vi "S3 Tool Initial.vi"() -> (0 "error constant":errorcluster)   [LabVIEW 2019]
uses:
  Ctrl/StationCmdSelect.ctl
  Ctrl/Auto Inspection Station Name2.ctl
  Ctrl/Auto Inspection Data Name.ctl
  Global/Process Global.vi
  LineScan/LineScan.lvclass
  LLB/Commonly VI.lvlib
panel:
  out "ToolStringOut_Init":string
  out "Initial_ChkSum":string
  out "S3 Initial Status":bool
  out "Initial receive":string
  out "retry次數 2":string[](array[string])
  out "CurrentCmd 2":string
  out "Retry 2":i32
  in  "Numeric 3":i32
  out "Act Step":i32
  out "Numeric":dbl
  out "subarray":string[](array[string])
  in  "error in (no error) 2":errorcluster
  out "retry次數":string[](array[string])
  out "CurrentCmd":string
  out "Retry":i32
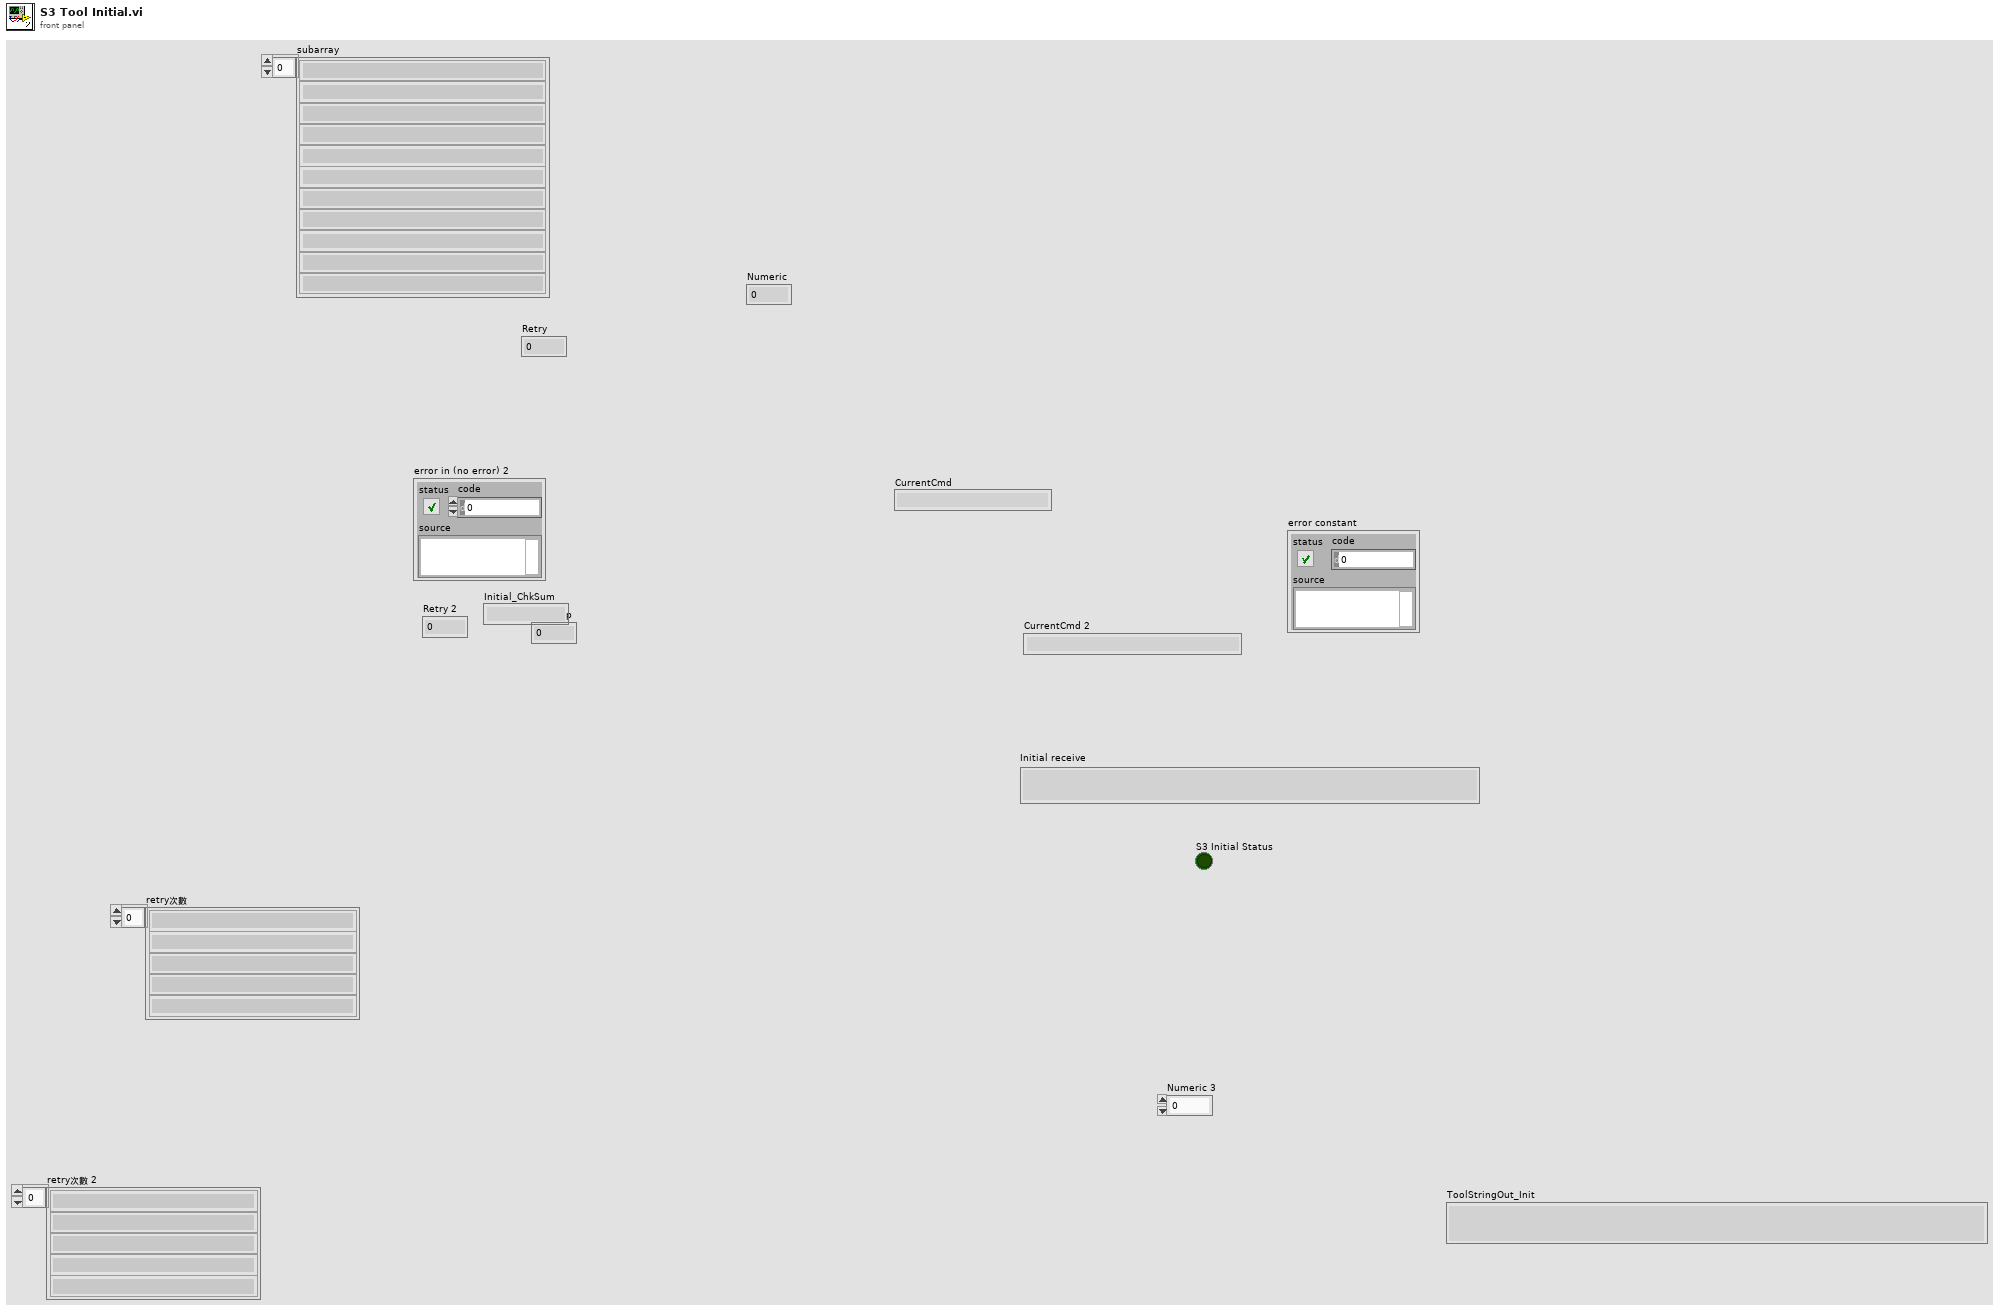
[diagram p1: front panel]
types:
  T1 = typedef "StationCmdSelect.ctl" = enum16{"Action", "Command", "Return", "DTime", "Retry"}
  T2 = typedef "Auto Inspection Data Name.ctl" = enum16{"LocalRun", "ItemSN(TimeCode)", "CurrentAction", "Error", "Data", "OKNG", "電壓值", "電壓值判斷", "電流值", "電流值判斷", "Laser1 Data", "Laser2 Data", "Laser OKNG", "StationNO"}
  T3 = typedef "Auto Inspection Station Name2.ctl" = enum16{"S1Barcode", "S2Measure", "S3Measure", "S4Measure", "S5Measure", "S11_LaserCheck", "S8_Vision AI"}
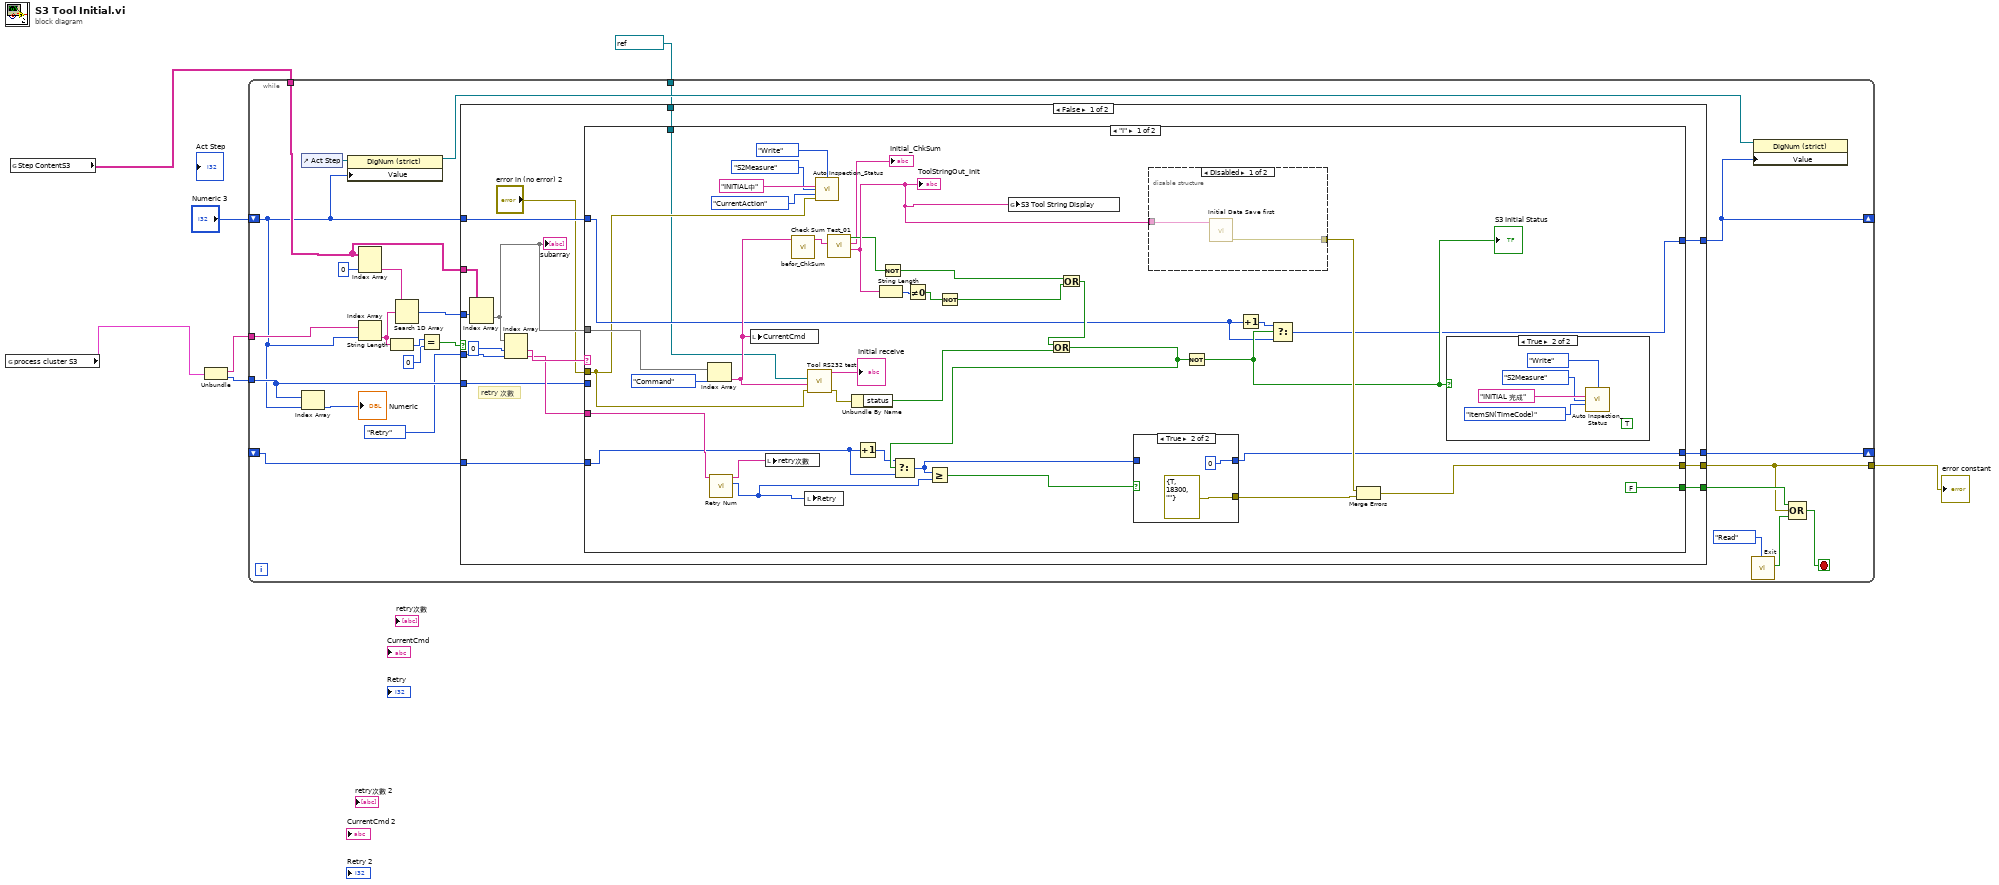
[diagram p0: block diagram]
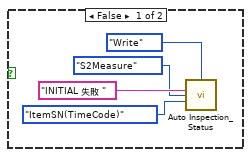
[diagram p3: hidden frame]
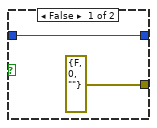
[diagram p4: hidden frame]
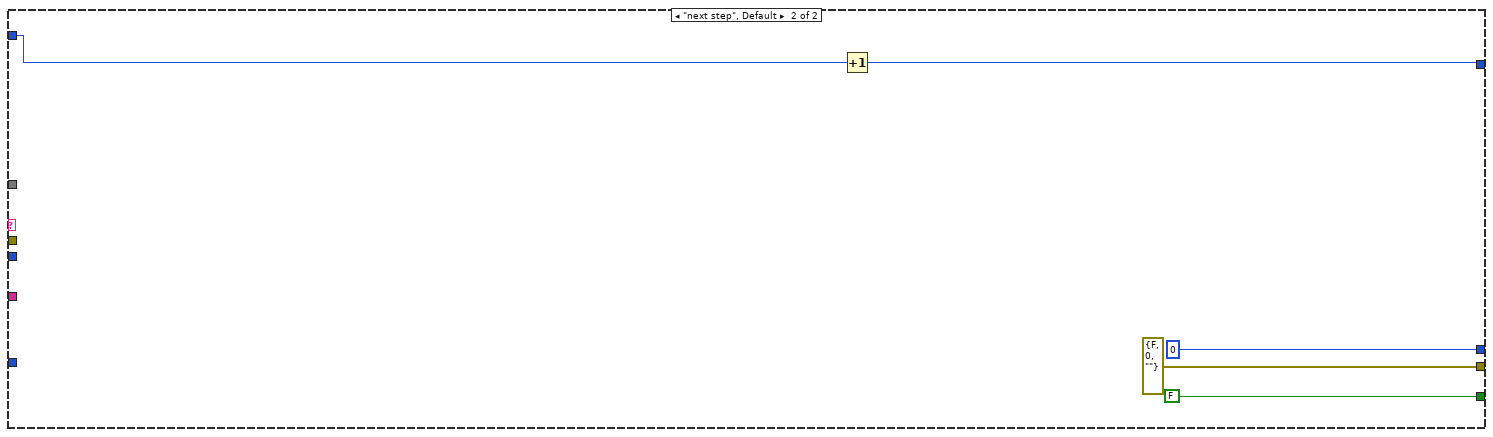
[diagram p5: hidden frame]
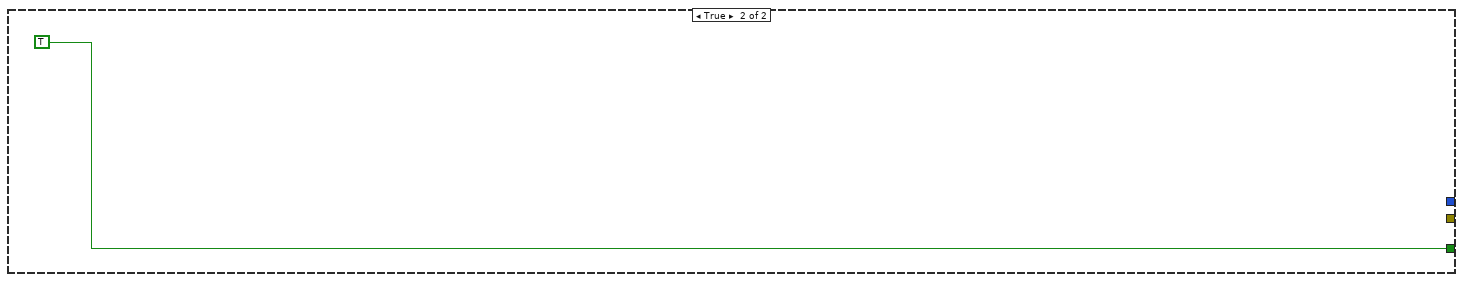
[diagram p6: hidden frame]
diagram:
  n1 = global read "Process Global.vi" "process cluster S3"() -> (w2:cluster{string[], i32[]})
  n2 = global read "Process Global.vi" "Step ContentS3"() -> (w3:string[][])
  n3 = Unbundle(w2) -> (w7:string[], w6:i32[])
  n4 = while {
    tunnel: w7 -> [w31]
    tunnel: w6 -> [w30]
    tunnel: w3 -> [w29]
    shift-right: [w14] -> _
    shift-left: _ -> [w18]
    shift-right: [w15] -> _
    shift-left: "Numeric 3" -> [w12]
    tunnel: [w11] -> w4
    tunnel: refnum<visa-resource-name> "COM3" ("VISA resource name") -> [w10]
    stop <- w19 stop-if-true
    n5 = control-ref of="Act Step"() -> (w17:refnum<vi>)
    n6 = Index Array(array=w30, index=w12) -> (element=→"Numeric":i32)
    n7 = property class="DigNum (strict)"(reference=w17, "Value"=w12) -> (reference out=w16:refnum<vi>)  [unwired: 1 in, 1 out]
    n8 = Index Array(array=w29, index (col)=0 ("disabled index (col)")) -> (element=w27:string[])  [unwired: 1 in]
    n9 = Index Array(array=w31, index=w12) -> (element=w24:string)
    n10 = String Length(string=w24) -> (length=w23:i32)
    n11 = Search 1D Array(1D array=w27, element=w24) -> (index of element=w26:i32)  [unwired: 1 in]
    n12 = Equal?(x=w23, y=0) -> (x = y?=w21:bool)
    n13 = case shown="False" w21 {
      tunnel: w29 -> [w47 _]
      tunnel: w26 -> [w46 _]
      tunnel: w30 -> [w42 _]
      tunnel: w18 -> [w40 _]
      tunnel: StationCmdSelect."Retry" -> [w39 _]
      tunnel: [w38 _] -> w11
      tunnel: w12 -> [w37 _]
      tunnel: [w36 _] -> w15
      tunnel: [w35 _] -> w14
      tunnel: [w34 TRUE] -> w13
      tunnel: w10 -> [w32 _]
      frame False {
        # "retry 次數"
        n14 = Index Array(array=w47, index (row)=w46) -> (element=w41:string[])  [unwired: 1 in]
        "subarray" <- w41
        n15 = Index Array(array=w41, index #1=0 ("index"), index #2=w39) -> (element #1=w44:string, element #2=w43:string)
        n16 = case shown="\"I\"" w44 {
          tunnel: w42 -> [_ _]
          tunnel: w43 -> [w53 _]
          tunnel: w41 -> [w55 _]
          tunnel: w40 -> [w52 _]
          tunnel: [w48 errorcluster {"status"=FALSE, "code"=0, "source"=""} ("error constant")] -> w38
          tunnel: w37 -> [w56 w104]
          tunnel: [w50 w103] -> w36
          tunnel: [w49 0] -> w35
          tunnel: [FALSE FALSE] -> w34
          tunnel: "error in (no error) 2" -> [w54 _]
          tunnel: w32 -> [w51 _]
          frame "I" {
            n17 = Index Array(array=w55, index=StationCmdSelect."Command") -> (element=w83:string)
            n18 = call "Retry Num.vi"("String"=w53) -> ("Numeric"=w84:i32, "retry次數"=w82:string[])  [unwired: 9 in]
            n19 = local write "CurrentCmd"(w83) -> ()
            n20 = local write "retry次數"(w82) -> ()
            n21 = call "befor_ChkSum.vi"("ToolString Input"=w83) -> ("Array"=w75:string[])  [unwired: 9 in, 1 out]
            n22 = local write "Retry"(w84) -> ()
            n23 = call "Tool RS232 test.vi"("error in (no error)"=w54, "Cmd In"=w83, "VISA resource name"=w51) -> ("error out"=w63:errorcluster, "receive string"=→"Initial receive":string)  [unwired: 7 in]
            n24 = call "Auto Inspection_Status.vi"("Action"=enum16{"Initial", "Write", "Read"}."Write", "DataIn"="INITIAL中", "Station"=Auto_Inspection_Station_Name2."S2Measure", "Data"=Auto_Inspection_Data_Name."CurrentAction", "error in"=w54) -> ()  [unwired: 8 in, 3 out]
            n25 = call "Check Sum Test_01.vi"("Array"=w75) -> ("ToolStringOut_01"=w80:string, "ChkSum"=→"Initial_ChkSum":string, "x = y?"=w78:bool)  [unwired: 8 in]
            "ToolStringOut_Init" <- w80
            n26 = Unbundle By Name(w63) -> ("status"=w68:bool)
            n27 = Increment(x=w52) -> (x+1=w62:i32)
            n28 = String Length(string=w80) -> (length=w72:i32)
            n29 = Not(x=w78) -> (.not. x?=w74:bool)
            n30 = Not Equal To 0?(x=w72) -> (x != 0?=w71:bool)
            n31 = Not(x=w71) -> (.not. x?=w73:bool)
            n32 = global write "Process Global.vi" "S3 Tool String Display"(w80) -> ()
            n33 = Or(x=w74, y=w73) -> (x .or. y?=w77:bool)
            n34 = Or(x=w77, y=w68) -> (x .or. y?=w69:bool)
            n35 = Select(t=w62, s=w69, f=w52) -> (s? t:f=w66:i32)
            n36 = Greater Or Equal?(x=w66, y=w84) -> (x >= y?=w64:bool)
            n37 = case shown="True" w64 {
              tunnel: [errorcluster {"status"=FALSE, "code"=0, "source"=""} ("error constant") errorcluster {"status"=TRUE, "code"=18300, "source"=""} ("error constant")] -> w79
              tunnel: w66 -> [w96 _]
              tunnel: [w96 0] -> w49
              frame False {
              }
              frame True {
              }
            }
            n38 = disable-structure shown="Disabled" {
              disable-tunnel: [w87 _] -> w81
              disable-tunnel: w80 -> [w86 _]
              frame Disabled {
                n39 = call "Initial Data Save first.vi"("String In"=w86) -> ("error out"=w87:errorcluster)  [unwired: 10 in]
              }
              frame Enabled {
              }
            }
            n40 = Not(x=w69) -> (.not. x?=w67:bool)
            "S3 Initial Status" <- w67
            n41 = Increment(x=w56) -> (x+1=w65:i32)
            n42 = Select(t=w65, s=w67, f=w56) -> (s? t:f=w50:i32)
            n43 = Merge Errors(w81, w79) -> (w48:errorcluster)
            n44 = case shown="True" w67 {
              frame False {
                n45 = call "Auto Inspection_Status.vi"("Action"=enum16{"Initial", "Write", "Read"}."Write", "DataIn"="INITIAL 失敗 ", "Station"=Auto_Inspection_Station_Name2."S2Measure", "Data"=Auto_Inspection_Data_Name."ItemSN(TimeCode)") -> ()  [unwired: 9 in, 3 out]
              }
              frame True {
                (unwired) TRUE
                n46 = call "Auto Inspection_Status.vi"("Action"=enum16{"Initial", "Write", "Read"}."Write", "DataIn"="INITIAL 完成", "Station"=Auto_Inspection_Station_Name2."S2Measure", "Data"=Auto_Inspection_Data_Name."ItemSN(TimeCode)") -> ()  [unwired: 9 in, 3 out]
              }
            }
          }
          frame "next step", Default {
            n47 = Increment(x=w104) -> (x+1=w103:i32)
          }
        }
      }
      frame True {
      }
    }
    n48 = call "Exit.vi"("Enum"=enum16{"Initial", "Read", "Write"}."Read") -> ("ExitOut"=w9:bool)  [unwired: 10 in]
    n49 = property class="DigNum (strict)"(reference=w16, "Value"=w15) -> ()  [unwired: 1 in, 2 out]
    n50 = Compound Arithmetic op=OR(w13, w11, w9) -> (w19:bool)
  }
  "error constant" <- w4
